vi "Set Space.vi"(8 "error in (no error)":errorcluster, 10 "Space":T1, 11 "Reversi in":refnum<class "Reversi.lvclass">) -> (0 "error out":errorcluster, 3 "Reversi out":refnum<class "Reversi.lvclass">)   [LabVIEW 2020, in "Reversi.lvlib" / "Reversi.lvclass"]
uses:
  Reversi.lvclass
  Space Cluster.ctl
  Space Coordinates.ctl
  Space Ring.ctl
  Reversi.lvclass/Reversi.ctl
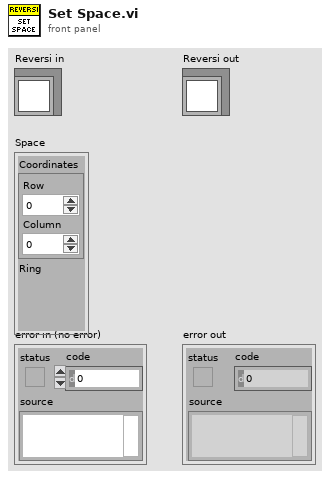
[diagram p1: front panel]
types:
  T1 = typedef "Reversi.lvlib/Reversi.lvclass/Space Cluster.ctl" = cluster{"Coordinates":T2, "Ring":T3}
  T2 = typedef "Reversi.lvlib/Reversi.lvclass/Space Coordinates.ctl" = cluster{"Row":i32, "Column":i32}
  T3 = typedef "Reversi.lvlib/Reversi.lvclass/Space Ring.ctl" = u16
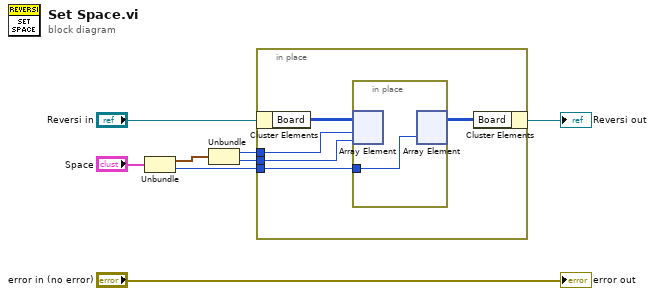
[diagram p0: block diagram]
diagram:
  n1 = Unbundle("Space") -> ("Coordinates"=w4:T2, "Ring"=w3:T3)
  n2 = Unbundle(w4) -> ("Row"=w2:i32, "Column"=w1:i32)
  n3 = in-place {
    in-place-border: w2 -> [w12]
    in-place-border: w1 -> [w11]
    in-place-border: w3 -> [w10]
    n4 = in-place-cluster #1("Reversi in") -> ("Board"=w13:T3[][])
    n5 = in-place {
      in-place-border: w10 -> [w14]
      n6 = in-place-array #2(w13, w12, w11) -> ()  [unwired: 1 out]
      n7 = in-place-array #2(w14) -> (w9:T3[][])  [unwired: 2 out]
    }
    n8 = in-place-cluster #1("Board"=w9) -> (→"Reversi out":refnum<class "Reversi.lvclass">)
  }
  "error out" <- "error in (no error)"
